vi "Decode_UnsignedHundredths.vi"(1 "Little Endian":u8[](array[numeric])) -> (0 "Unsigned Hundredths (0.00)":dbl[](array[numeric]))   [LabVIEW 2015, in "navX Library v3.lvlib" / "navX Registry Cache.lvclass"]
uses:
  navX Registry Cache.lvclass
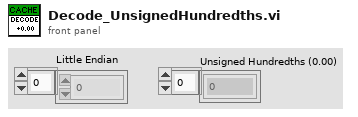
[diagram p1: front panel]
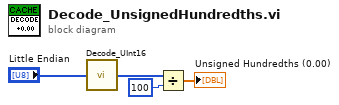
[diagram p0: block diagram]
diagram:
  n1 = call "Decode_UInt16.vi"("Little Endian"="Little Endian") -> ("UInt16"=w2:u16[])
  n2 = Divide(x=w2, y=100) -> (x/y=→"Unsigned Hundredths (0.00)":dbl[])
